vi "Waveform Acquisition - Write (1xI16).vi"(0 "data in":i16, 1 "reset":bool, 2 "Waveform Acquisition Resources":T2, 5 "input valid":bool, 11 "bypass DRAM FIFO (F)":bool, 12 "latch utilization":bool) -> (3 "reset done":bool, 10 "memory utilization":T1, 14 "ready for input":bool, 15 "FIFO utilization":T1)   [LabVIEW 2018, in "Streaming FPGA.lvlib"]
doc: "Waveform Acquisition control and writer.\n\nThe Waveform Acquisition streams a waveform to the host through a DRAM FIFO.\n\nThe resources for the Waveform Acquisition must be created by the <B>Waveform Acquisition - Create Resources.vi</B>. The Waveform Acquisition also requires the <B>Waveform Acquisition - Process.vi</B> to be placed on the block diagram and to be connected to the <B>Waveform Acquisition - Create Resources.vi</B>. Both of those VIs must be placed on the block diagram outside of any SCTLs.\n\nThis VI must be placed inside an SCTL.\n\nInputs:\n\n<B>Waveform Acquisition Resources</B>: Input for the Waveform Acquisition resources. Connect the <B>Waveform Acquisition - Create Resources.vi</B> output to this input.\n\n<B>data in</B>: Data input, this input is an I16.\n\n<B>input valid</B>: A true on this input signals that the <B>data in</B> input is valid. The data input is processed by this VI if the <B>ready for input</B> output was true in the previous cycle.\n\n<B>bypass DRAM FIFO</B>: A true on this input disables the use of the <B>DRAM Memory</B> memory element. The Waveform Acquisition can buffer at least 16*(<B>DRAM Memory Size</B>+1024) I16 elements in case the DRAM is enabled (the <B>bypass DRAM FIFO</B> input is false), and 16*1024 I16 elements in case the DRAM is disabled (<B>bypass DRAM FIFO</B> is true). <B>DRAM Memory Size</B> is the requested number of elements parameter of the memory resource (provided on the <B>Waveform Acquisition - Create Resources.vi</B> input).\n\n<B>reset</B>: A true on this input resets the Waveform Acquisition.\n\n<B>latch utilization</B>: A rising edge on this input updates the <B>memory utilization</B> and <B>FIFO utilization</B> outputs in the next cycle and starts a new utilization tracking period.\n\nOutputs:\n\n<B>reset done</B>: A true on the <B>reset</B> input sets this output to false, the completion of the reset cycle is signaled by this output becoming true.\n\n<B>ready for input</B>: A true on this output signals that this VI will be ready for data input in the next cycle.\n\n<B>memory utilization</B>: Is the <B>lowest</B> and <B>highest</B> number of I16 elements waited in the Waveform Acquisition during the previous utilization tracking period. A new tracking period can be started by creating a rising edge on the <B>latch utilization</B> input. The utilization period starts automatically each time a reset cycle is complete.\n\n<B>FIFO utilization</B>: Is the <B>lowest</B> and <B>highest</B> number of I16 elements waited in the input FIFO accepting the data input during the previous utilization tracking period. A new tracking period can be started by creating a rising edge on the <B>latch utilization</B> input. The utilization period starts automatically each time a reset cycle is complete.\n\nFollow these steps to initialize the Waveform Acquisition:\n\n1. Stop writing the data input of this VI.\n2. Set the <B>reset</B> input to true, then set to false.\n3. Wait until the <B>reset done</B> output becomes true.\n4. Clear the <B>T2H FIFO</B> specified on the <B>Waveform Acquisition - Create Resources.vi</B> input (use the Start and Stop FIFO interface methods on the Host).\n5. Start writing the data input of this VI."
uses:
  Streaming FPGA.lvlib
  Waveform Acquisition Resources (1xI16).ctl
  Target-Scoped FIFO (1xI16) Resource.ctl
  FIFO Utilization.ctl
  <vilib>/rvi/DataTransferAndStorage/Container/Common/niFpgaContainerExecOnDevCompGetState.vi
  <vilib>/rvi/Emulation/niFpgaEmulationIsFPGAContextNoSignature.vi
  <vilib>/rvi/DataTransferAndStorage/Container/Common/niFpgaContainerGetUniqueNameForEmu.vi
  <vilib>/rvi/Memory/Memory_Emulation/niFpgaMemoryEmulationCacheClearOnFirstRun.vi
  <vilib>/rvi/Memory/Memory_Emulation/nirvimemoryEmulationManagerCache_MakeExclusive.vi
  <vilib>/rvi/Memory/Memory_Emulation/niFpgaMemoryEmulationValidateCache.vi
  <vilib>/rvi/Memory/Memory_Emulation/nirvimemoryEmulationManagerCache_InsertValue.vi
  <vilib>/Utility/error.llb/Clear Errors.vi
  <vilib>/rvi/Memory/Memory_Emulation/nirvimemoryEmulationManagerCache_ReleaseExclusive.vi
  <vilib>/rvi/Memory/Memory_Emulation/nirvimemoryEmulationManagerCache_GetValue.vi
  <vilib>/rvi/Memory/Memory_Emulation/nirvimemoryEmulationManagerCache_SetValue.vi
  <vilib>/rvi/Emulation/niFpgaProcessEmulError.vi
  <vilib>/rvi/Emulation/niFpgaSctlEmulationGetInTimedLoop.vi
  <instrlib>/_niInstr/Basic Elements/v1/FPGA/Private/Count Up U32.vi
  <vilib>/rvi/DataTransferAndStorage/Container/XNode/niFpgaContainer.xnode
  <vilib>/rvi/DataTransferAndStorage/Register/Emulation/niFpgaRegisterEmulationRefIn.vi
  <instrlib>/_niInstr/Basic Elements/v1/FPGA/niInstr Basic Elements v1 FPGA.lvlib
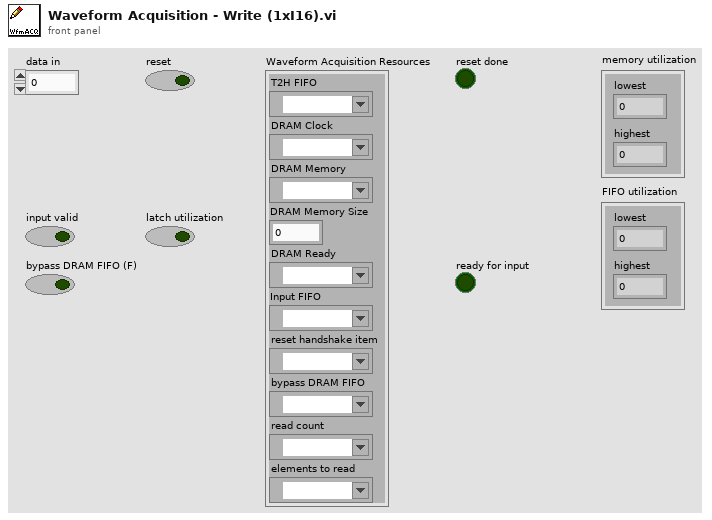
[diagram p1: front panel]
types:
  T1 = typedef "Streaming FPGA.lvlib/FIFO Utilization.ctl" = cluster{"lowest":u32, "highest":u32}
  T2 = typedef "Streaming FPGA.lvlib/Waveform Acquisition Resources (1xI16).ctl" = cluster{"T2H FIFO":refnum<k21>, "DRAM Clock":refnum<k21>, "DRAM Memory":refnum<k21>, "DRAM Memory Size":u32, "DRAM Ready":refnum<k21>, "Input FIFO":T3, "reset handshake item":refnum<k21>, "bypass DRAM FIFO":refnum<k21>, "read count":refnum<k21>, "elements to read":refnum<k21>}
  T3 = typedef "Streaming FPGA.lvlib/Target-Scoped FIFO (1xI16) Resource.ctl" = refnum<k21>
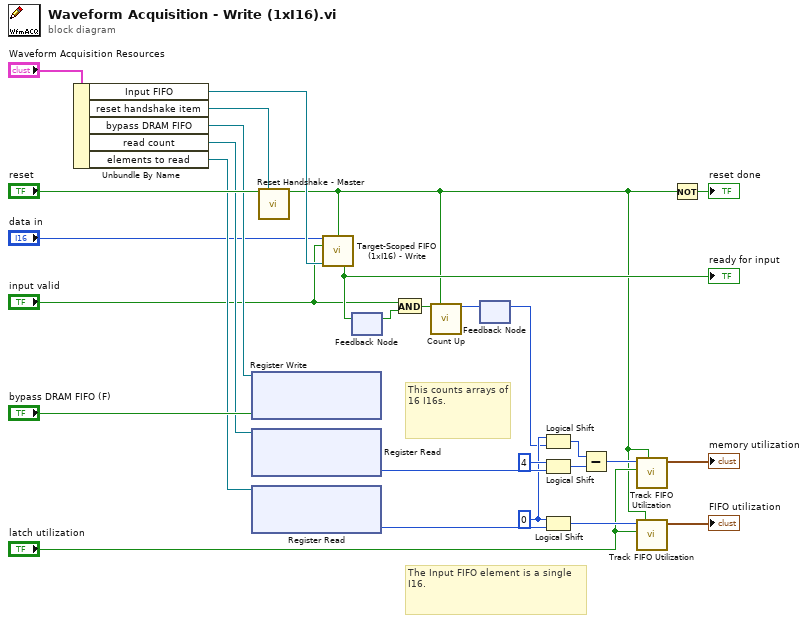
[diagram p0: block diagram]
diagram:
  w10 = i16 0 ("y")
  # "This counts arrays of 16 I16s."
  # "The Input FIFO element is a single I16."
  n1 = Unbundle By Name("Waveform Acquisition Resources") -> ("Input FIFO"=w25:T3, "reset handshake item"=w26:refnum<k21>, "bypass DRAM FIFO"=w23:refnum<k21>, "read count"=w21:refnum<k21>, "elements to read"=w20:refnum<k21>)
  n2 = xnode "Register Write"("Data"="bypass DRAM FIFO (F)", "Register In"=w23) -> ()  [unwired: 1 out]
  n3 = xnode "Register Read"("Register In"=w21) -> ("Data"=w14:u32)  [unwired: 1 out]
  n4 = xnode "Register Read"("Register In"=w20) -> ("Data"=w11:u32)  [unwired: 1 out]
  n5 = call "Reset Handshake - Master.vi"("reset in"="reset", "reset handshake item"=w26) -> ("reset out"=w4:bool)  [unwired: 13 in]
  n6 = call "Target-Scoped FIFO (1xI16) - Write.vi"("data in"="data in", "reset"=w4, "input valid"="input valid", "Target-Scoped FIFO (1xI16)"=w25) -> ("ready for input"=w19:bool)  [unwired: 10 in, 1 out]
  "ready for input" <- w19
  n7 = feedback-in #1(w19) -> ()
  n8 = feedback #1() -> (w18:bool)  [unwired: 1 in]
  n9 = And(x="input valid", y=w18) -> (x .and. y?=w16:bool)
  n10 = call-poly <instrlib>:"Count Up.vi"("increment"=w16, "reset"=w4) -> ("count out"=w3:u32)  [unwired: 13 in]
  n11 = feedback-in #2(w3) -> ()
  n12 = feedback #2() -> (w2:u32)  [unwired: 1 in]
  n13 = Logical Shift(y=w10, x=w2) -> (x << y=w13:u32)
  n14 = Logical Shift(y=i16 4, x=w14) -> (x << y=w12:u32)
  n15 = Logical Shift(y=w10, x=w11) -> (x << y=w7:u32)
  n16 = Subtract(x=w13, y=w12) -> (x-y=w9:u32)
  n17 = call "Track FIFO Utilization.vi"("reset"=w4, "latch utilization"="latch utilization", "samples available"=w9) -> ("FIFO utilization"=→"memory utilization":T1)  [unwired: 8 in]
  n18 = call "Track FIFO Utilization.vi"("reset"=w4, "latch utilization"="latch utilization", "samples available"=w7) -> ("FIFO utilization"=→"FIFO utilization":T1)  [unwired: 8 in]
  n19 = Not(x=w4) -> (.not. x?=→"reset done":bool)
